vi "start server accept.vi"(5 "id":u32, 7 "event":refnum<user-event>, 8 "error in":errorcluster, 11 "acceptor":u64) -> (0 "error out":errorcluster)   [LabVIEW 2016, in "async tls.lvlib"]
uses:
  async tls.lvlib
  tls new socket user event.ctl
  lvasynctls.dll
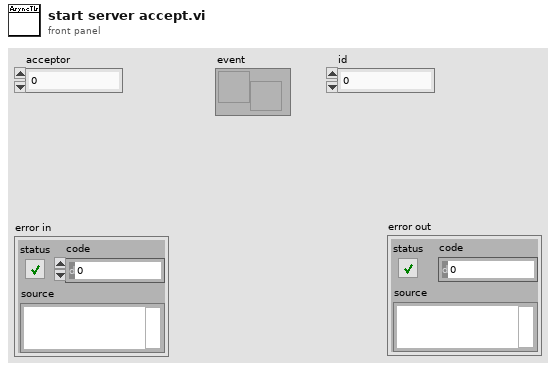
[diagram p1: front panel]
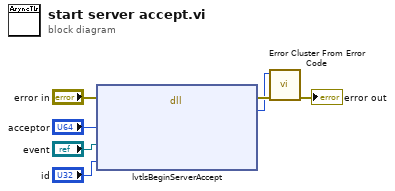
[diagram p0: block diagram]
diagram:
  n1 = dll-call lib="C:/Users/IEUser/Desktop/libasynclvtls/lvasynctls.dll" fn="lvtlsBeginServerAccept"(error in="error in", "acceptor"="acceptor", "event"="event", "id"="id") -> (error out=w3:errorcluster, "err"=w1:i32)  [unwired: 5 in, 1 out]
  n2 = call <vilib>:"Error Cluster From Error Code.vi"("error in (no error)"=w3, "error code (0)"=w1) -> ("error out"=→"error out":errorcluster)  [unwired: 7 in]
